vi "Follower.vi"() -> ()   [LabVIEW 2016]
uses:
  <vilib>/NXT/Block Support/NXT_InputPort.ctl
  <vilib>/NXT/Block Support/NXT_TimerIndex.ctl
  <vilib>/NXT/Block Support/NXT_OutputPort.ctl
  <vilib>/NXT/Dual Mode Library/Sensors/EV3_Gyro_Reset.vi
  <vilib>/NXT/Dual Mode Library/Sensors/EV3_Gyro_Angle.vi
  <vilib>/NXT/Dual Mode Library/Sensors/EV3_Gyro_Rate.vi
  <vilib>/NXT/Dual Mode Library/Sensors/Reset_Timer.vi
  <vilib>/NXT/Dual Mode Library/Sensors/EV3_Color_Reflect.vi
  <vilib>/NXT/Dual Mode Library/Sensors/Read_Timer.vi
  <vilib>/NXT/Dual Mode Library/Sensors/EV3_Ultrasonic_CM.vi
  <vilib>/NXT/Dual Mode Library/Display/drawText_Right.vi
  <vilib>/NXT/Dual Mode Library/prims/inRangeAndCoerce/inRangeAndCoerce_float.vi
  <vilib>/NXT/NXTIO Xnodes/NXTIONodeSubVIs/NXTMoveMotors.vi
  <vilib>/NXT/Dual Mode Library/Display/drawNumber.vi
  <vilib>/NXT/Dual Mode Library/Display/drawNumber_float.vi
  <vilib>/NXT/Dual Mode Library/Motors/Rotation.vi
  <vilib>/NXT/Dual Mode Library/Motors/ResetMotor.vi
  <vilib>/NXT/Dual Mode Library/Sound/Tone.vi
  <vilib>/NXT/Dual Mode Library/Display/drawText.vi
  <vilib>/NXT/NXTIO Xnodes/NXTIONodeSubVIs/NXTStopMotors.vi
  <vilib>/NXT/Subs/LVHSConnector.ctl
  <vilib>/NXT/NXTIO Xnodes/AddressXNode/NXTIOAddress.xnode
  <vilib>/NXT/NXTIO Xnodes/NXTIOXNode/NXTIO.xnode
  <vilib>/NXT/LegoClasses/BrickReference/BrickReference.lvclass
panel:
  out "Value (msec)":u32
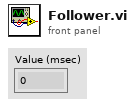
[diagram p1: front panel]
types:
  T1 = typedef "NXT_InputPort.ctl" = u32
  T2 = typedef "LVHSConnector.ctl" = refnum<class "BrickReference.lvclass">
  T3 = typedef "NXT_TimerIndex.ctl" = u8
  T4 = typedef "NXT_OutputPort.ctl" = u8
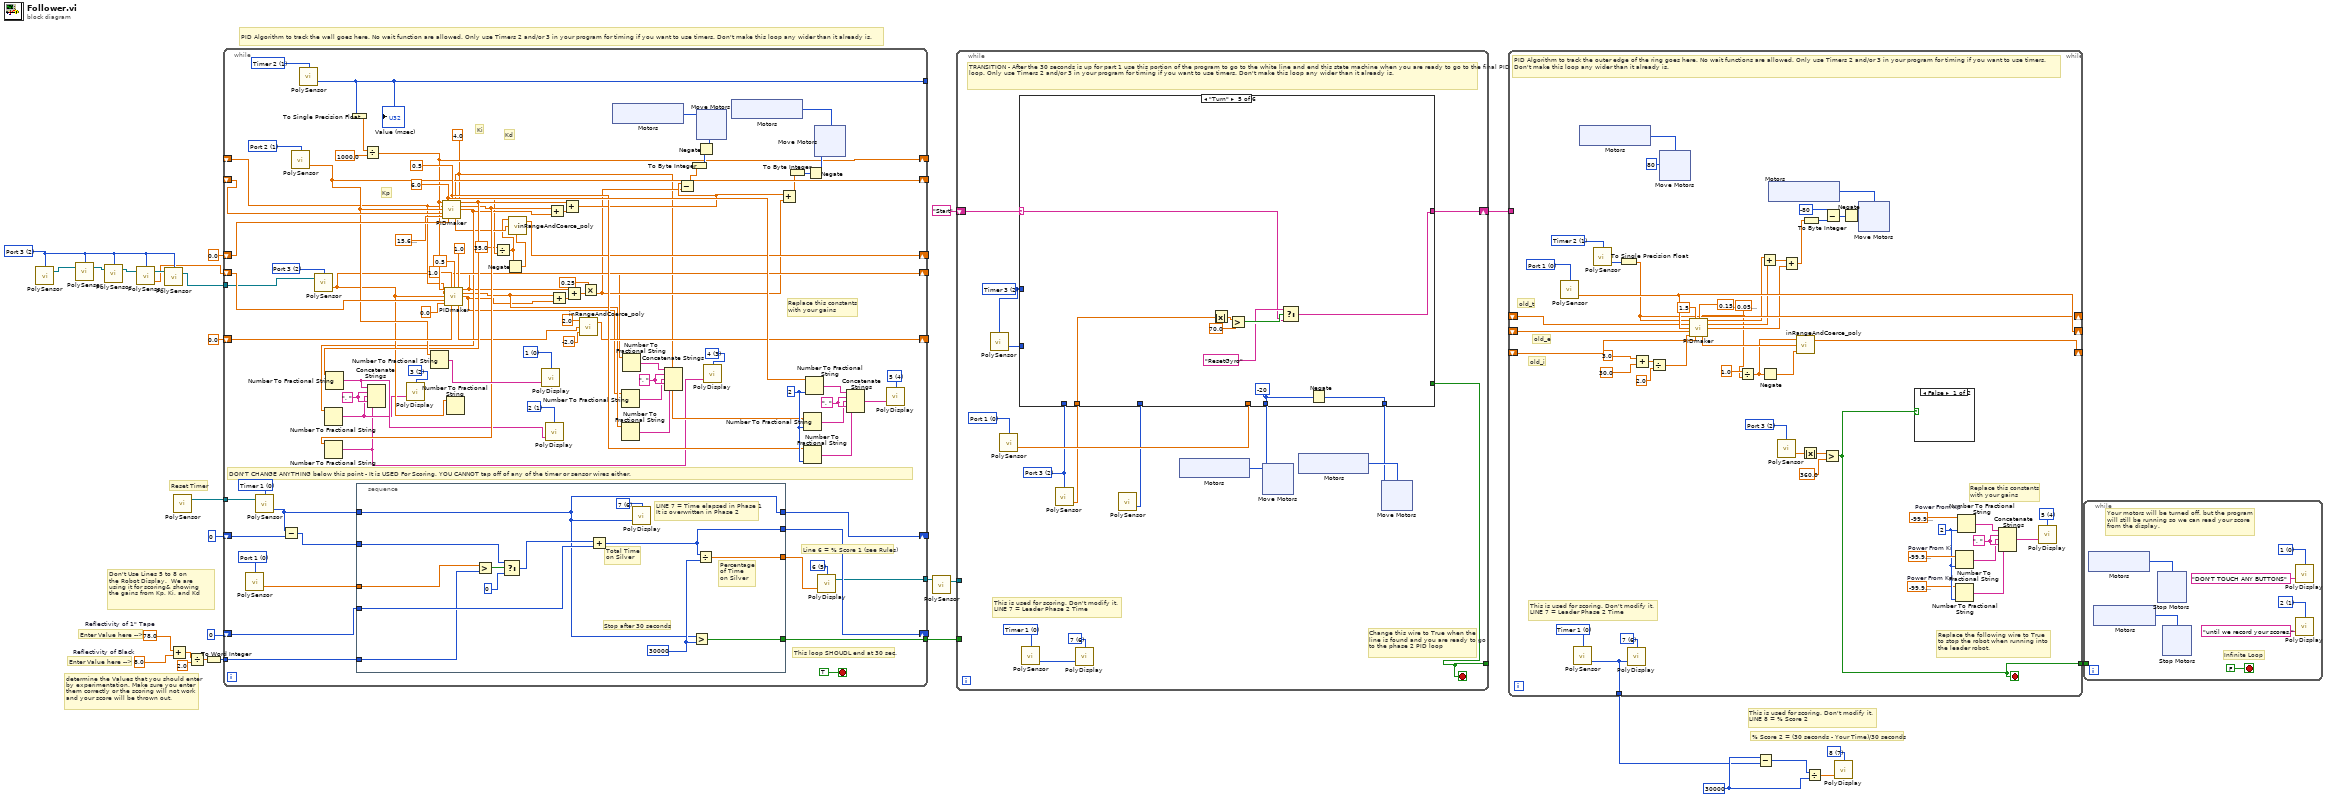
[diagram p0: block diagram]
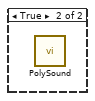
[diagram p2: hidden frame]
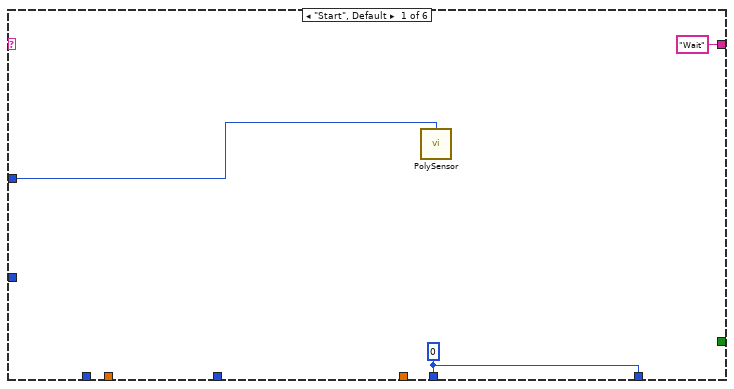
[diagram p3: hidden frame]
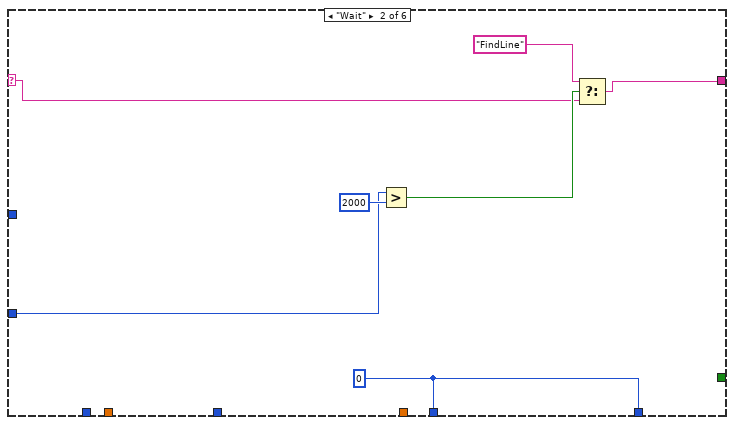
[diagram p4: hidden frame]
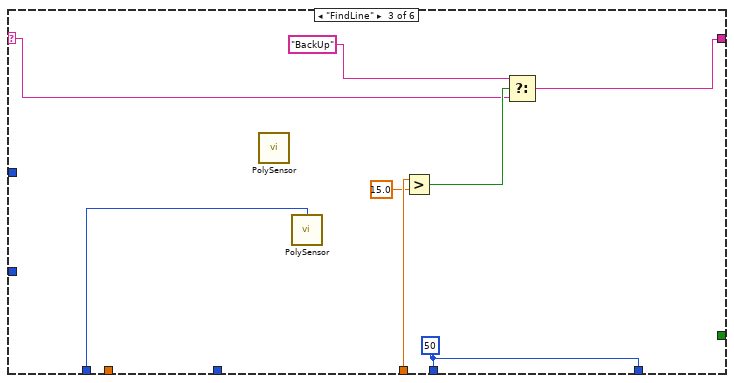
[diagram p5: hidden frame]
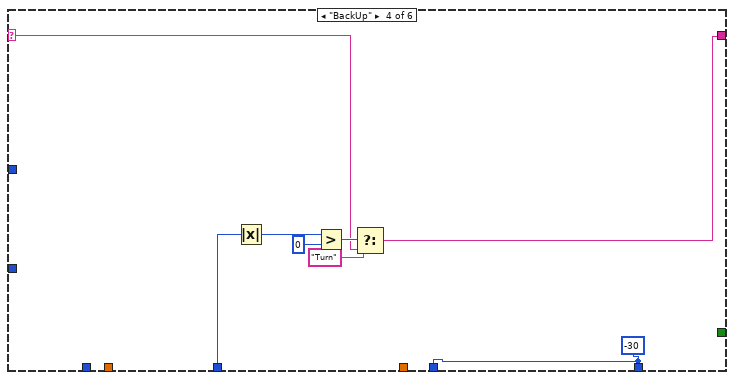
[diagram p6: hidden frame]
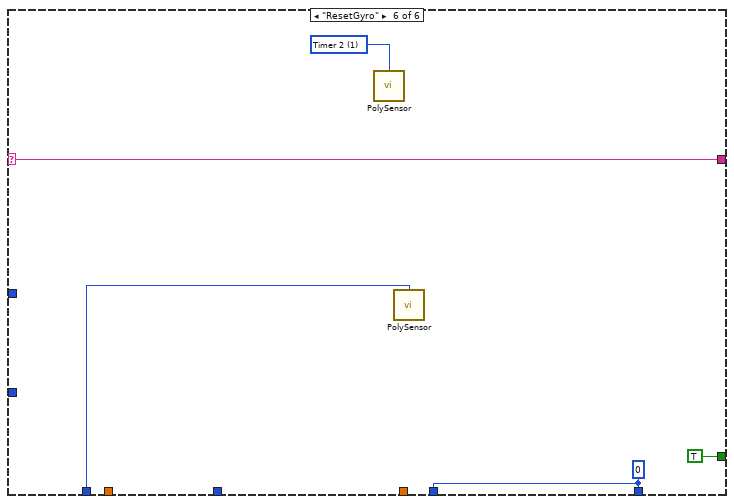
[diagram p7: hidden frame]
diagram:
  w5 = T1 2 items=["Port 1", "Port 2", "Port 3", "Port 4"] ("Port (Port 1)")
  w13 = u32 30000 ("Value (msec)")
  w14 = i16 7 items=["1", "2", "3", "4", "5", "6", "7", "8", "9", "10", "11", "12"] ("Line")
  w20 = 8.0  # Reflectivity of Black
  w19 = 78.0  # Reflectivity of 1" Tape
  # "PID Algorithm to track the wall goes here. No wait function are allowed. Only use Timers 2 and/or 3 in your program for timing if you want to use timers. Don't make this loop any wider than it already is."
  # "This is used for scoring. Don't modify it.\nLINE 8 = % Score 2"
  # "Don't Use Lines 5 to 8 on\nthe Robot Display.  We are \nusing it for scoring& showing \nthe gains from Kp, Ki, and Kd"
  # "% Score 2 = (30 seconds - Your Time)/30 seconds"
  # "Enter Value here -->"
  # "determine the Values that you should enter\nby experimentation. Make sure you enter \nthem correctly or the scoring will not work\nand your score will be thrown out."
  # "Enter Value here -->"
  # "Reset Timer"
  n1 = call-poly <vilib>:"PolySensor.vi"("Port (Port 1)"=w5) -> ("NXT/EV3"=w6:T2)  [unwired: 3 in]
  n2 = call-poly <vilib>:"PolySensor.vi"("NXT/EV3"=w6, "Port (Port 1)"=w5) -> ("NXT/EV3"=w7:T2)  [unwired: 1 in, 1 out]
  n3 = call-poly <vilib>:"PolySensor.vi"("NXT/EV3"=w7, "Port (Port 1)"=w5) -> ("NXT/EV3"=w9:T2)  [unwired: 1 in, 1 out]
  n4 = call-poly <vilib>:"PolySensor.vi"("NXT/EV3"=w9, "Port (Port 1)"=w5) -> ("Degrees"=w1:sgl, "NXT/EV3"=w8:T2)  [unwired: 1 in]
  n5 = call-poly <vilib>:"PolySensor.vi"("NXT/EV3"=w8, "Port (Port 1)"=w5) -> ("NXT/EV3"=w4:T2)  [unwired: 2 in]
  n6 = Add(x=w19, y=w20) -> (x+y=w18:dbl)
  n7 = call-poly <vilib>:"PolySensor.vi"() -> ("NXT/EV3"=w27:T2)  [unwired: 4 in]
  n8 = Divide(x=w18, y=2.0) -> (x/y=w17:dbl)
  n9 = To Word Integer(number=w17) -> (16bit integer=w24:i16)
  n10 = while {
    shift-right: [w113] -> _
    shift-left: i16 0 -> [w117]
    shift-right: [w114] -> _
    shift-left: i16 0 ("Value (msec)") -> [w116]
    tunnel: w27 -> [w112]
    tunnel: [w115] -> w26
    tunnel: w24 -> [w107]
    tunnel: [w103] -> w22
    shift-right: [w48] -> _
    shift-left: sgl 0.0 ("coerced(x)") -> [w84]
    shift-right: [w63] -> _
    shift-left: sgl 0.0 ("coerced(x)") -> [w89]
    shift-right: [w52] -> _
    shift-left: w1 -> [w87]
    tunnel: [w83] -> _
    shift-right: [w58] -> _
    shift-left: _ -> [w57]
    shift-right: [w71] -> _
    shift-left: _ -> [w79]
    tunnel: w4 -> [w51]
    stop <- TRUE stop-if-true
    w44 = ", " ("string")
    w41 = i16 3 items=["1", "2", "3", "4", "5", "6", "7", "8", "9", "10", "11", "12"] ("Line")
    w53 = i16 1 items=["1", "2", "3", "4", "5", "6", "7", "8", "9", "10", "11", "12"] ("Line")
    w70 = ", " ("string")
    w69 = i16 2 items=["1", "2", "3", "4", "5", "6", "7", "8", "9", "10", "11", "12"] ("Line")
    w73 = i16 0 items=["1", "2", "3", "4", "5", "6", "7", "8", "9", "10", "11", "12"] ("Line")
    w37 = sgl 4.0 ("Ki")
    w76 = sgl 0.5 ("Kd")
    w77 = sgl 6.0 ("Kp")
    w80 = T1 1 items=["Port 1", "Port 2", "Port 3", "Port 4"] ("Port (Port 1)")
    w85 = T3 1 items=["Timer 1", "Timer 2", "Timer 3"] ("Timer (Timer 1)")
    w88 = T1 2 items=["Port 1", "Port 2", "Port 3", "Port 4"] ("Port (Port 1)")
    w99 = ", " ("string")
    w101 = i16 2 ("precision (6)")
    w102 = i16 4 items=["1", "2", "3", "4", "5", "6", "7", "8", "9", "10", "11", "12"] ("Line")
    w105 = i16 5 items=["1", "2", "3", "4", "5", "6", "7", "8", "9", "10", "11", "12"] ("Line")
    w109 = T1 0 items=["Port 1", "Port 2", "Port 3", "Port 4"] ("Port (Port 3)")
    w110 = T3 0 items=["Timer 1", "Timer 2", "Timer 3"] ("Timer (Timer 1)")
    # "Kp"
    # "Kd"
    # "Ki"
    # "Replace this constants\nwith your gains"
    # "DON'T CHANGE ANYTHING below this point - It is USED For Scoring. YOU CANNOT tap off of any of the timer or sensor wires either."
    # "Line 6 = % Score 1 (see Rules)"
    # "This loop SHOUDL end at 30 sec."
    n11 = call-poly <vilib>:"PolySensor.vi"("Port (Port 1)"=w109) -> ("Scaled Value"=w108:sgl)  [unwired: 2 in, 1 out]
    n12 = call-poly <vilib>:"PolySensor.vi"("NXT/EV3"=w112, "Timer (Timer 1)"=w110) -> ("Value (msec)"=w111:u32)  [unwired: 1 in, 1 out]
    n13 = Subtract(x=w111, y=w116) -> (x-y=w106:u32)
    n14 = call-poly <vilib>:"PolySensor.vi"("Port (Port 1)"=w80) -> ("Centimeters"=w71:sgl)  [unwired: 2 in, 1 out]
    n15 = call-poly <vilib>:"PolySensor.vi"("Timer (Timer 1)"=w85) -> ("Value (msec)"=w83:u32)  [unwired: 2 in, 1 out]
    "Value (msec)" <- w83
    n16 = call-poly <vilib>:"PolySensor.vi"("NXT/EV3"=w51, "Port (Port 1)"=w88) -> ("Degrees"=w52:sgl)  [unwired: 1 in, 1 out]
    n17 = To Single Precision Float(number=w83) -> (single precision float=w81:sgl)
    n18 = stacked-sequence {
      tunnel: w117 -> [w146]
      tunnel: [w136] -> w104
      tunnel: w111 -> [w134]
      tunnel: [w145] -> w115
      tunnel: w108 -> [w140]
      tunnel: w106 -> [w142]
      tunnel: [w134] -> w114
      tunnel: [w138] -> w113
      tunnel: w107 -> [w139]
      frame #0 {
        w135 = i16 6 items=["1", "2", "3", "4", "5", "6", "7", "8", "9", "10", "11", "12"] ("Line")
        w137 = u32 30000 ("Value (msec)")
        # "LINE 7 = Time elapsed in Phase 1\nIt is overwritten in Phase 2"
        # "Percentage\nof Time\non Silver"
        # "Stop after 30 seconds"
        # "Total Time\non Silver"
        n19 = Greater?(x=w140, y=w139) -> (0:w143:bool)
        n20 = Select(t=w142, s=w143, f=i16 0) -> (s? t:f=w141:u32)
        n21 = Add(x=w141, y=w146) -> (x+y=w138:u32)
        n22 = call-poly <vilib>:"PolyDisplay.vi"("number"=w134, "Line"=w135) -> ()  [unwired: 2 in, 1 out]
        n23 = Greater?(x=w134, y=w137) -> (0:w145:bool)
        n24 = Divide(x=w138, y=w137) -> (x/y=w136:dbl)
      }
    }
    n25 = Divide(x=w81, y=sgl 1000.0) -> (x/y=w58:sgl)
    n26 = Number To Fractional String(number=w71) -> (F-format string=w72:string)  [unwired: 3 in]
    n27 = call "PIDmaker.vi"("New Time"=w58, "Kp"=w77, "Kd"=w76, "Ki"=w37, "Old Time"=w57, "New Value"=w71, "Old Value"=w79, "Desired Value"=sgl 15.6, "Integral In"=w84) -> ("P out"=w68:sgl, "D out"=w67:sgl, "I out"=w50:sgl, "Integral Out"=w49:sgl)  [unwired: 3 in]
    n28 = Number To Fractional String(number=w50) -> (F-format string=w32:string)  [unwired: 3 in]
    n29 = Number To Fractional String(number=w67) -> (F-format string=w31:string)  [unwired: 3 in]
    n30 = Number To Fractional String(number=w68) -> (F-format string=w33:string)  [unwired: 3 in]
    n31 = Concatenate Strings(w33, w70, w32, w70, w31) -> ()  [unwired: 1 out]
    n32 = call-poly <vilib>:"PolyDisplay.vi"("Text"=w32, "Line"=w69) -> ()  [unwired: 2 in, 1 out]
    n33 = call "PIDmaker.vi"("New Time"=w58, "Kp"=sgl 1.0, "Kd"=sgl 0.5, "Ki"=sgl 1.0, "Old Time"=w57, "New Value"=w52, "Old Value"=w87, "Desired Value"=sgl 0.0, "Integral In"=w89) -> ("P out"=w40:sgl, "D out"=w39:sgl, "I out"=w38:sgl, "Integral Out"=w64:sgl)  [unwired: 3 in]
    n34 = Number To Fractional String(number=w52) -> ()  [unwired: 3 in, 1 out]
    n35 = Divide(x=sgl 35.0, y=w37) -> (x/y=w35:sgl)
    n36 = Negate(x=w35) -> (-x=w34:sgl)
    n37 = call-poly <vilib>:"inRangeAndCoerce_poly.vi"("lower limit"=w34, "x"=w49, "upper limit"=w35) -> ("coerced(x)"=w48:sgl)  [unwired: 1 out]
    n38 = call-poly <vilib>:"PolyDisplay.vi"("Text"=w72, "Line"=w73) -> ()  [unwired: 2 in, 1 out]
    n39 = call-poly <vilib>:"PolyDisplay.vi"("Text"=w33, "Line"=w53) -> ()  [unwired: 2 in, 1 out]
    n40 = Add(x=w67, y=w50) -> (x+y=w93:sgl)
    n41 = Add(x=w39, y=w38) -> (x+y=w90:sgl)
    n42 = Add(x=w68, y=w93) -> (x+y=w61:sgl)
    n43 = Add(x=w40, y=w90) -> (x+y=w59:sgl)
    n44 = call-poly <vilib>:"inRangeAndCoerce_poly.vi"("lower limit"=sgl -2.0, "x"=w64, "upper limit"=sgl 2.0) -> ("coerced(x)"=w63:sgl)  [unwired: 1 out]
    n45 = Multiply(x=sgl 0.25, y=w59) -> (x*y=w47:sgl)
    n46 = xnode "Motors"() -> ("Motor"=w95:T4)
    n47 = Number To Fractional String(number=w38) -> (F-format string=w43:string)  [unwired: 3 in]
    n48 = Number To Fractional String(number=w39) -> (F-format string=w42:string)  [unwired: 3 in]
    n49 = Number To Fractional String(number=w40) -> (F-format string=w45:string)  [unwired: 3 in]
    n50 = Concatenate Strings(w45, w44, w43, w44, w42) -> ()  [unwired: 1 out]
    n51 = Subtract(x=w61, y=w47) -> (x-y=w62:sgl)
    n52 = To Byte Integer(number=w62) -> (8bit integer=w74:i8)
    n53 = Negate(x=w74) -> (-x=w66:i8)
    n54 = xnode "Move Motors"("Power/Speed 1"=w66, "Motors"=w95) -> ()  [unwired: 1 in, 1 out]
    n55 = call-poly <vilib>:"PolyDisplay.vi"("Text"=w31, "Line"=w41) -> ()  [unwired: 2 in, 1 out]
    n56 = xnode "Motors"() -> ("Motor"=w94:T4)
    n57 = Add(x=w61, y=w47) -> (x+y=w60:sgl)
    n58 = To Byte Integer(number=w60) -> (8bit integer=w75:i8)
    n59 = Number To Fractional String(number=w37, precision (6)=w101) -> (F-format string=w98:string)  [unwired: 2 in]
    n60 = Number To Fractional String(number=w76, precision (6)=w101) -> (F-format string=w97:string)  [unwired: 2 in]
    n61 = Number To Fractional String(number=w77, precision (6)=w101) -> (F-format string=w100:string)  [unwired: 2 in]
    n62 = Negate(x=w75) -> (-x=w65:i8)
    n63 = xnode "Move Motors"("Power/Speed 1"=w65, "Motors"=w94) -> ()  [unwired: 1 in, 1 out]
    n64 = call-poly <vilib>:"PolyDisplay.vi"("number"=w104, "Line"=w105) -> ("NXT/EV3"=w103:T2)  [unwired: 2 in]
    n65 = Concatenate Strings(w100, w99, w98, w99, w97) -> (w96:string)
    n66 = call-poly <vilib>:"PolyDisplay.vi"("Text"=w96, "Line"=w102) -> ()  [unwired: 2 in, 1 out]
  }
  n67 = call-poly <vilib>:"PolySensor.vi"("NXT/EV3"=w22) -> ("NXT/EV3"=w21:T2)  [unwired: 3 in]
  n68 = while {
    tunnel: w26 -> [_]
    shift-right: [w162] -> w15
    shift-left: "Start" -> [w163]
    tunnel: w21 -> [_]
    tunnel: [w147] -> _
    stop <- w147 stop-if-true
    w150 = T1 2 items=["Port 1", "Port 2", "Port 3", "Port 4"] ("Port (Port 1)")
    w152 = T1 0 items=["Port 1", "Port 2", "Port 3", "Port 4"] ("Port (Port 1)")
    w156 = T3 2 items=["Timer 1", "Timer 2", "Timer 3"] ("Timer (Timer 1)")
    w159 = i16 6 items=["1", "2", "3", "4", "5", "6", "7", "8", "9", "10", "11", "12"] ("Line")
    w161 = T3 0 items=["Timer 1", "Timer 2", "Timer 3"] ("Timer (Timer 1)")
    # "This is used for scoring. Don't modify it.\nLINE 7 = Leader Phase 2 Time"
    # "Change this wire to True when the line is found and you are ready to go to the phase 2 PID loop"
    # "TRANSITION - After the 30 seconds is up for part 1 use this portion of the program to go to the white line and end this state machine when you are ready to go to the final PID control loop. Only use Timers 2 and/or 3 in your program for timing if you want to use timers. Don't make this loop any wider than it already is."
    n69 = call-poly <vilib>:"PolySensor.vi"("Timer (Timer 1)"=w156) -> ("Value (msec)"=w155:u32)  [unwired: 2 in, 1 out]
    n70 = call-poly <vilib>:"PolySensor.vi"("Port (Port 1)"=w152) -> ("Scaled Value"=w151:sgl)  [unwired: 2 in, 1 out]
    n71 = call-poly <vilib>:"PolySensor.vi"("Timer (Timer 1)"=w161) -> ("Value (msec)"=w160:u32)  [unwired: 2 in, 1 out]
    n72 = call-poly <vilib>:"PolySensor.vi"("Port (Port 1)"=w150) -> ("Degrees"=w149:sgl)  [unwired: 2 in, 1 out]
    n73 = call-poly <vilib>:"PolyDisplay.vi"("number"=w160, "Line"=w159) -> ()  [unwired: 2 in, 1 out]
    n74 = call-poly <vilib>:"PolySensor.vi"() -> ("Angle of Rotation"=w148:i32)  [unwired: 3 in, 1 out]
    n75 = case shown="\"Turn\"" w163 {
      selector: w163 -> [_ w185 w192 w200 w207 w217]
      tunnel: ["Wait" w188 w194 w198 w206 w217] -> w162
      tunnel: w156 -> [w182 _ _ _ _ _]
      tunnel: w155 -> [_ w184 _ _ _ _]
      tunnel: [w180 w183 w190 w205 w214 w216] -> w154
      tunnel: [w180 w183 w190 w205 w213 w216] -> w153
      tunnel: w151 -> [_ _ w197 _ _ _]
      tunnel: w150 -> [_ _ w191 _ _ w219]
      tunnel: w149 -> [_ _ _ _ w212 _]
      tunnel: w148 -> [_ _ _ w204 _ _]
      tunnel: [_ _ _ _ _ TRUE] -> w147
      frame "Start", Default {
        w180 = 0
        n76 = call-poly <vilib>:"PolySensor.vi"("Timer (Timer 1)"=w182) -> ()  [unwired: 3 in, 1 out]
      }
      frame "Wait" {
        w183 = 0
        n77 = Greater?(x=w184, y=u32 2000) -> (0:w186:bool)
        n78 = Select(t="FindLine", s=w186, f=w185) -> (s? t:f=w188:string)
      }
      frame "FindLine" {
        w190 = 50
        n79 = call-poly <vilib>:"PolySensor.vi"() -> ()  [unwired: 4 in, 1 out]
        n80 = call-poly <vilib>:"PolySensor.vi"("Port (Port 1)"=w191) -> ()  [unwired: 3 in, 1 out]
        n81 = Greater?(x=w197, y=sgl 15.0) -> (0:w195:bool)
        n82 = Select(t="BackUp", s=w195, f=w192) -> (s? t:f=w194:string)
      }
      frame "BackUp" {
        w205 = -30
        n83 = Absolute Value(x=w204) -> (abs(x)=w202:i32)
        n84 = Greater?(x=w202, y=0) -> (0:w201:bool)
        n85 = Select(t="Turn", s=w201, f=w200) -> (s? t:f=w198:string)
      }
      frame "Turn" {
        w214 = -20
        n86 = Absolute Value(x=w212) -> (abs(x)=w211:sgl)
        n87 = Greater?(x=w211, y=sgl 70.0) -> (0:w209:bool)
        n88 = Select(t="ResetGyro", s=w209, f=w207) -> (s? t:f=w206:string)
        n89 = Negate(x=w214) -> (-x=w213:i32)
      }
      frame "ResetGyro" {
        w215 = T3 1 items=["Timer 1", "Timer 2", "Timer 3"] ("Timer (Timer 1)")
        w216 = 0
        n90 = call-poly <vilib>:"PolySensor.vi"("Timer (Timer 1)"=w215) -> ()  [unwired: 3 in, 1 out]
        n91 = call-poly <vilib>:"PolySensor.vi"("Port (Port 1)"=w219) -> ()  [unwired: 3 in, 1 out]
      }
    }
    n92 = xnode "Motors"() -> ("Motor"=w158:T4)
    n93 = xnode "Move Motors"("Power/Speed 1"=w154, "Motors"=w158) -> ()  [unwired: 1 in, 1 out]
    n94 = xnode "Motors"() -> ("Motor"=w157:T4)
    n95 = xnode "Move Motors"("Power/Speed 1"=w153, "Motors"=w157) -> ()  [unwired: 1 in, 1 out]
  }
  n96 = while {
    tunnel: [w220] -> w16
    tunnel: w15 -> [_]
    tunnel: [w268] -> w12
    shift-right: [w253] -> _
    shift-left: _ -> [w252]
    shift-right: [w249] -> _
    shift-left: _ -> [w248]
    shift-right: [w236] -> _
    shift-left: _ -> [w237]
    stop <- w220 stop-if-true
    w224 = T1 2 items=["Port 1", "Port 2", "Port 3", "Port 4"] ("Port (Port 1)")
    w234 = sgl 0.06 ("Ki")
    w255 = T3 1 items=["Timer 1", "Timer 2", "Timer 3"] ("Timer (Timer 1)")
    w256 = T1 0 items=["Port 1", "Port 2", "Port 3", "Port 4"] ("Port (Port 1)")
    w261 = ", " ("string")
    w264 = i16 2 ("precision (6)")
    w263 = sgl -99.9  # Power From Kd
    w265 = sgl -99.9  # Power From Ki
    w266 = sgl -99.9  # Power From Kp
    w267 = i16 4 items=["1", "2", "3", "4", "5", "6", "7", "8", "9", "10", "11", "12"] ("Line")
    w269 = i16 6 items=["1", "2", "3", "4", "5", "6", "7", "8", "9", "10", "11", "12"] ("Line")
    w270 = T3 0 items=["Timer 1", "Timer 2", "Timer 3"] ("Timer (Timer 1)")
    # "old_i"
    # "old_e"
    # "old_t"
    # "Replace this constants\nwith your gains"
    # "This is used for scoring. Don't modify it.\nLINE 7 = Leader Phase 2 Time"
    # "PID Algorithm to track the outer edge of the ring goes here. No wait functions are allowed. Only use Timers 2 and/or 3 in your program for timing if you want to use timers.\nDon't make this loop any wider than it already is."
    # "Replace the following wire to True\nto stop the robot when running into \nthe leader robot."
    n97 = call-poly <vilib>:"PolySensor.vi"("Port (Port 1)"=w256) -> ("Scaled Value"=w253:sgl)  [unwired: 2 in, 1 out]
    n98 = call-poly <vilib>:"PolySensor.vi"("Timer (Timer 1)"=w270) -> ("Value (msec)"=w268:u32)  [unwired: 2 in, 1 out]
    n99 = xnode "Motors"() -> ("Motor"=w230:T4)
    n100 = call-poly <vilib>:"PolySensor.vi"("Timer (Timer 1)"=w255) -> ("Value (msec)"=w254:u32)  [unwired: 2 in, 1 out]
    n101 = To Single Precision Float(number=w254) -> (single precision float=w249:sgl)
    n102 = call-poly <vilib>:"PolyDisplay.vi"("number"=w268, "Line"=w269) -> ()  [unwired: 2 in, 1 out]
    n103 = Add(x=sgl 3.0, y=sgl 30.0) -> (x+y=w247:sgl)
    n104 = Divide(x=w247, y=sgl 2.0) -> (x/y=w244:sgl)
    n105 = xnode "Move Motors"("Power/Speed 1"=i8 80, "Motors"=w230) -> ()  [unwired: 1 in, 1 out]
    n106 = call "PIDmaker.vi"("New Time"=w249, "Kp"=sgl 1.5, "Kd"=sgl 0.15, "Ki"=w234, "Old Time"=w248, "New Value"=w253, "Old Value"=w252, "Desired Value"=w244, "Integral In"=w237) -> ("P out"=w240:sgl, "D out"=w239:sgl, "I out"=w238:sgl, "Integral Out"=w243:sgl)  [unwired: 3 in]
    n107 = Divide(x=sgl 1.0, y=w234) -> (x/y=w232:sgl)
    n108 = Add(x=w240, y=w239) -> (x+y=w241:sgl)
    n109 = Negate(x=w232) -> (-x=w233:sgl)
    n110 = xnode "Motors"() -> ("Motor"=w257:T4)
    n111 = call-poly <vilib>:"PolySensor.vi"("Port (Port 1)"=w224) -> ("Degrees"=w223:sgl)  [unwired: 2 in, 1 out]
    n112 = Add(x=w241, y=w238) -> (x+y=w231:sgl)
    n113 = call-poly <vilib>:"inRangeAndCoerce_poly.vi"("lower limit"=w233, "x"=w243, "upper limit"=w232) -> ("coerced(x)"=w236:sgl)  [unwired: 1 out]
    n114 = Absolute Value(x=w223) -> (abs(x)=w221:sgl)
    n115 = To Byte Integer(number=w231) -> (8bit integer=w228:i8)
    n116 = Greater?(x=w221, y=sgl 360.0) -> (0:w220:bool)
    n117 = Subtract(x=i8 -80, y=w228) -> (x-y=w226:i8)
    n118 = Negate(x=w226) -> (-x=w225:i8)
    n119 = xnode "Move Motors"("Power/Speed 1"=w225, "Motors"=w257) -> ()  [unwired: 1 in, 1 out]
    n120 = case shown="False" w220 {
      frame False {
      }
      frame True {
        n121 = call-poly <vilib>:"PolySound.vi"() -> ()  [unwired: 4 in, 1 out]
      }
    }
    n122 = Number To Fractional String(number=w265, precision (6)=w264) -> (F-format string=w260:string)  [unwired: 2 in]
    n123 = Number To Fractional String(number=w263, precision (6)=w264) -> (F-format string=w259:string)  [unwired: 2 in]
    n124 = Number To Fractional String(number=w266, precision (6)=w264) -> (F-format string=w262:string)  [unwired: 2 in]
    n125 = Concatenate Strings(w262, w261, w260, w261, w259) -> (w258:string)
    n126 = call-poly <vilib>:"PolyDisplay.vi"("Text"=w258, "Line"=w267) -> ()  [unwired: 2 in, 1 out]
  }
  n127 = Subtract(x=w13, y=w12) -> (x-y=w11:u32)
  n128 = Divide(x=w11, y=w13) -> (x/y=w10:dbl)
  n129 = call-poly <vilib>:"PolyDisplay.vi"("number"=w10, "Line"=w14) -> ()  [unwired: 2 in, 1 out]
  n130 = while {
    tunnel: w16 -> [_]
    stop <- FALSE stop-if-true
    w287 = i16 1 items=["1", "2", "3", "4", "5", "6", "7", "8", "9", "10", "11", "12"] ("Line")
    w290 = i16 0 items=["1", "2", "3", "4", "5", "6", "7", "8", "9", "10", "11", "12"] ("Line")
    # "Your motors will be turned off, but the program\nwill still be running so we can read your score\nfrom the display."
    # "Infinite Loop"
    n131 = xnode "Motors"() -> ("Motor"=w292:T4)
    n132 = xnode "Motors"() -> ("Motor"=w291:T4)
    n133 = xnode "Stop Motors"("Motors"=w292) -> ()  [unwired: 1 in, 1 out]
    n134 = xnode "Stop Motors"("Motors"=w291) -> ()  [unwired: 1 in, 1 out]
    n135 = call-poly <vilib>:"PolyDisplay.vi"("Text"="DON'T TOUCH ANY BUTTONS", "Line"=w290) -> ()  [unwired: 2 in, 1 out]
    n136 = call-poly <vilib>:"PolyDisplay.vi"("Text"="until we record your scores.", "Line"=w287) -> ()  [unwired: 2 in, 1 out]
  }
